vi "SUBLTdll.vi"(8 "error in (no error)":errorcluster, 11 "Inputs":cluster{"t":dbl, "z":dbl[], "p":dbl}) -> (0 "error out":errorcluster, 3 "Outputs":T1)   [LabVIEW 2016]
doc: "subroutine SUBLTdll(t, z, p, ierr, herr, herr_length)\n\nCompute the sublimation line pressure as a function of temperature and composition.\n\nINPUTS:\nt -- Temperature [K]\nz -- Composition (array of mole fractions)\n\nOUTPUTS:\np -- Sublimation line pressure [kPa] ierr, herr: See error codes in the ANCERR1 routine.\nierr -- error flag: 0 = successful\nherr -- error string\nherr_length -- length of variable herr (default: 255)"
uses:
  REFPROP.DLL
panel:
  # "REFPROP-SUBLTdll.vi"
  # "void  SUBLTdll(double *t, double *z, double *p, int32_t *ierr, CStr herr, int32_t herr_length)"
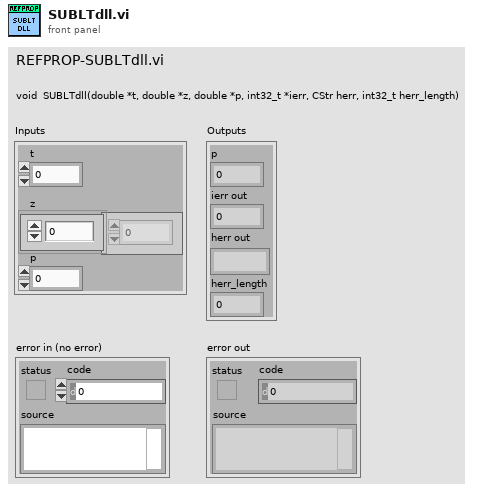
[diagram p1: front panel]
types:
  T1 = cluster{"p ":dbl, "ierr out":i32, "herr out":string, "herr_length":i32}
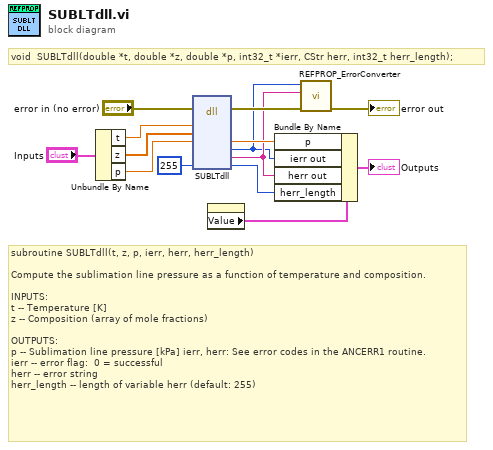
[diagram p0: block diagram]
diagram:
  # "void  SUBLTdll(double *t, double *z, double *p, int32_t *ierr, CStr herr, int32_t herr_length);"
  # "subroutine SUBLTdll(t, z, p, ierr, herr, herr_length)\n\nCompute the sublimation line pressure as a function of temperature and composition.\n\nINPUTS:\nt -- Temperature [K]\nz -- Composition (array of mole fractions)\n\nOUTPUTS:\np -- Sublimation line pressure [kPa] ierr, herr: See error codes in the ANCERR1 routine.\nierr -- error flag:  0 = successful\nherr -- error string\nherr_length -- length of variable herr (default: 255)"
  n1 = Unbundle By Name("Inputs") -> ("t"=w6:dbl, "z"=w7:dbl[], "p"=w8:dbl)
  n2 = dll-call lib="S:/009 - Testing/02 - Performance Testing/REFPROP/REFPROP.*" fn="SUBLTdll"(error in="error in (no error)", "t"=w6, "z"=w7, "p"=w8, "herr_length"=255 ("ln")) -> (error out=w13:errorcluster, "p"=w3:dbl, "ierr"=w1:i32, "herr"=w2:string, "herr_length"=w4:i32)  [unwired: 7 in, 1 out]
  n3 = property on="Outputs" class="Clust (strict)"() -> ("Value"=w5:T1)  [unwired: 2 in, 2 out]
  n4 = Bundle By Name(cluster=w5, "p"=w3, "ierr out"=w1, "herr out"=w2, "herr_length"=w4) -> (→"Outputs":T1)
  n5 = call "REFPROP_ErrorConverter.vi"("error in (no error)"=w13, "Error Message"=w2, "Error Code"=w1) -> ("error out"=→"error out":errorcluster)  [unwired: 8 in]
